vi "Handle Error.vi"(8 "error in (no error)":errorcluster, 11 "UI ActorTop in":refnum<class "UI_Top.lvclass">) -> (0 "error out":errorcluster, 2 "stop actor?":bool=TRUE, 3 "UI ActorTop out":refnum<class "UI_Top.lvclass">)   [LabVIEW 2021, in "UI_Top.lvclass"]
doc: "(<B>Filename</B>: Actor Framework.lvlib:Actor.lvclass:Handle Error.vi)\n\nDefines how the actor handles an error that occurred while processing a message. By default, this method does nothing except stop the actor."
uses:
  UI_Top.lvclass
  UI_Top.lvclass/UI_Top.ctl
  <userlib>/John_Lib/AbstractActorTemplate/AbstractActorTemplate/UIActorTop.lvclass
  <vilib>/ActorFramework/Stop Msg/Stop Msg.lvclass
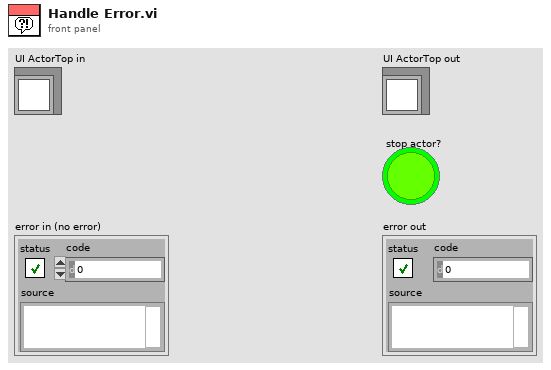
[diagram p1: front panel]
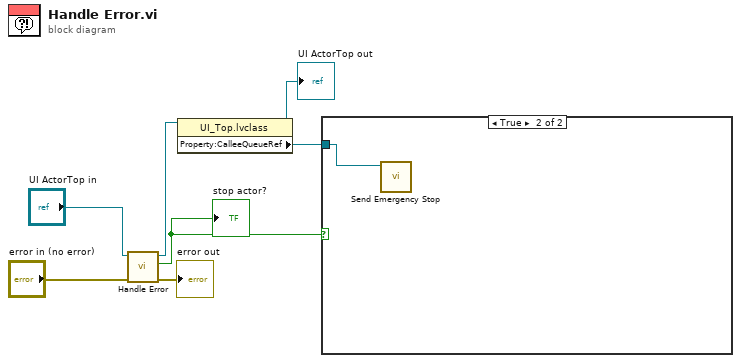
[diagram p0: block diagram]
diagram:
  n1 = call-parent "Handle Error.vi"("error in (no error)"="error in (no error)", "UI ActorTop in"="UI ActorTop in") -> ("error out"=→"error out":errorcluster, "stop actor?"=w3:bool, "UI ActorTop out"=w6:refnum<class "UI_Top.lvclass">)  [unwired: 7 in]
  "stop actor?" <- w3
  n2 = property class="UI_Top.lvclass"(reference=w6) -> (reference out=→"UI ActorTop out":refnum<class "UI_Top.lvclass">, "Property:CalleeQueueRef"=w1:refnum<class "Message Enqueuer.lvclass">)  [unwired: 1 in, 1 out]
  n3 = case shown="True" w3 {
    tunnel: w1 -> [_ w8]
    frame False {
    }
    frame True {
      n4 = call <vilib>:"Send Emergency Stop.vi"("Message Enqueuer"=w8) -> ()  [unwired: 10 in, 1 out]
    }
  }
